vi "Append schedule.vi"(8 "error in (no error)":errorcluster, 10 "Schedule to append":refnum<class "Schedule.lvclass">, 11 "Schedule in":refnum<class "Schedule.lvclass">) -> (0 "error out":errorcluster, 3 "Schedule out":refnum<class "Schedule.lvclass">)   [LabVIEW 2020, in "TALOS.lvlib" / "Run Utilities.lvlib" / "Schedule.lvclass"]
doc: "Combine two schedules into one. The VI checks if the last script of the schedule is the same as the first script of the appended one. If so, it combines two cells into one."
uses:
  Schedule.lvclass
  Cell/Schedule Cell.lvclass
  Schedule.lvclass/Schedule.ctl
  995fc32b-001c-43f1-ab01-1b4acc13e53d.vi
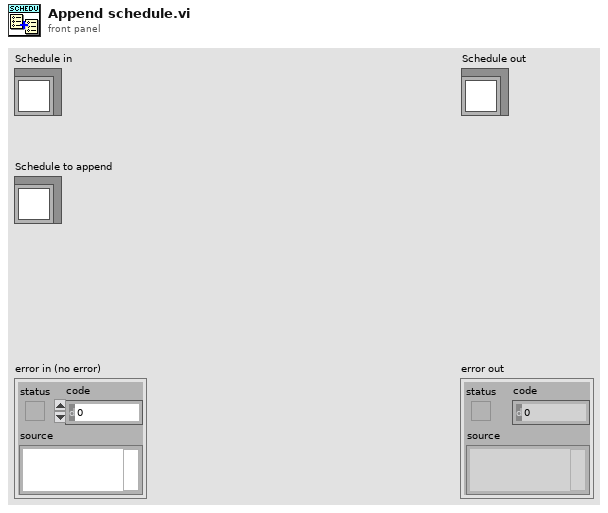
[diagram p1: front panel]
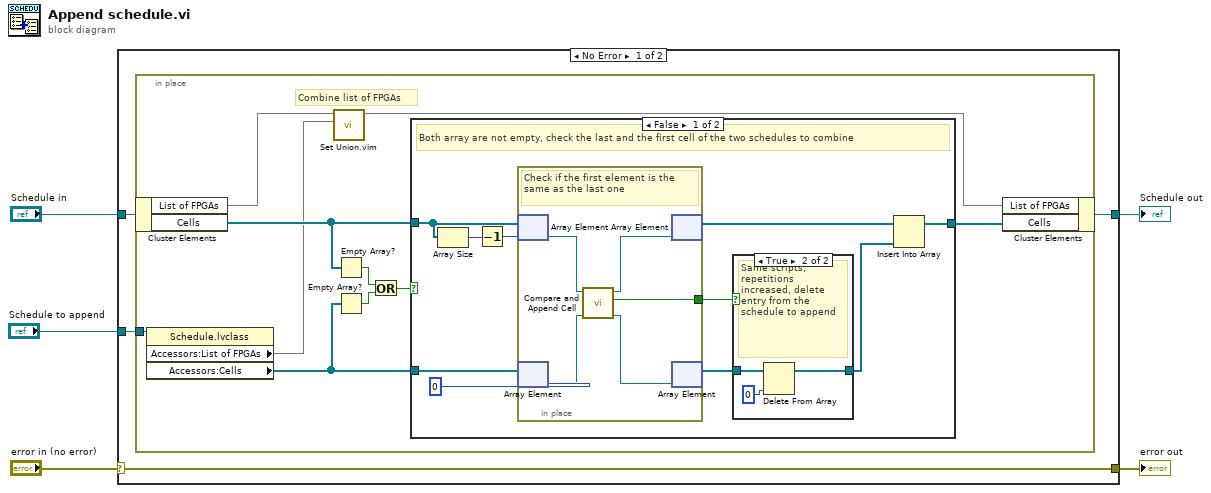
[diagram p0: block diagram]
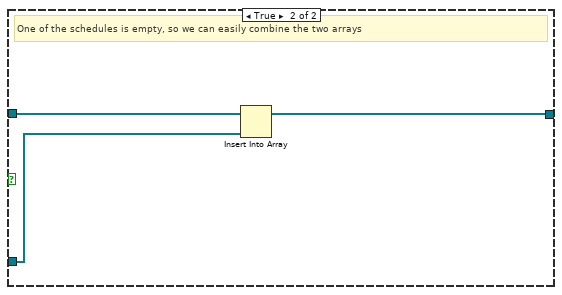
[diagram p3: hidden frame]
diagram:
  n1 = case shown="No Error" "error in (no error)" {
    selector: "error in (no error)" -> [w9 w43]
    tunnel: [w9 w43] -> w4
    tunnel: [w6 w42] -> w2
    tunnel: "Schedule in" -> [w7 w42]
    tunnel: "Schedule to append" -> [w8 _]
    frame No Error {
      n2 = in-place {
        in-place-border: w8 -> [w19]
        # "Combine list of FPGAs"
        n3 = in-place-cluster #1(w7) -> ("List of FPGAs"=w12:set{string}, "Cells"=w18:refnum<class "Schedule Cell.lvclass">[])
        n4 = property class="Schedule.lvclass"(reference=w19) -> ("Accessors:List of FPGAs"=w11:set{string}, "Accessors:Cells"=w16:refnum<class "Schedule Cell.lvclass">[])  [unwired: 1 in, 2 out]
        n5 = call "Set Union.vim"("set 2"=w11, "set 1"=w12) -> ("union"=w10:set{string})  [unwired: 9 in]
        n6 = Empty Array?(array=w18) -> (empty?=w15:bool)
        n7 = Empty Array?(array=w16) -> (empty?=w14:bool)
        n8 = Or(x=w15, y=w14) -> (x .or. y?=w13:bool)
        n9 = case shown="False" w13 {
          tunnel: [w20 w39] -> w17
          tunnel: w18 -> [w29 w41]
          tunnel: w16 -> [w28 w40]
          frame False {
            # "Both array are not empty, check the last and the first cell of the two schedules to combine"
            n10 = Array Size(array=w29) -> (size(s)=w27:i32)
            n11 = Decrement(x=w27) -> (x-1=w26:i32)
            n12 = in-place {
              in-place-border: [w32] -> w24
              # "Check if the first element is the same as the last one"
              n13 = in-place-array #2(w29, w26) -> (w31:refnum<class "Schedule Cell.lvclass">)
              n14 = in-place-array #3(w28, 0) -> (w30:refnum<class "Schedule Cell.lvclass">)
              n15 = call-dynamic "Compare and Append Cell.vi"("Schedule Cell B in"=w30, "Schedule Cell A in"=w31) -> ("Schedule Cell B out"=w33:refnum<class "Schedule Cell.lvclass">, "Cell Updated"=w32:bool, "Schedule Cell A out"=w34:refnum<class "Schedule Cell.lvclass">)  [unwired: 7 in]
              n16 = in-place-array #2(w34) -> (w21:refnum<class "Schedule Cell.lvclass">[])  [unwired: 1 out]
              n17 = in-place-array #3(w33) -> (w23:refnum<class "Schedule Cell.lvclass">[])  [unwired: 1 out]
            }
            n18 = case shown="True" w24 {
              tunnel: w23 -> [w35 w38]
              tunnel: [w35 w36] -> w22
              frame False {
                # "Not the same, do nothing"
              }
              frame True {
                # "Same scripts, repetitions increased, delete entry from the schedule to append"
                n19 = Delete From Array(array=w38, index=0) -> (array with subset deleted=w36:refnum<class "Schedule Cell.lvclass">[])  [unwired: 1 in, 1 out]
              }
            }
            n20 = Insert Into Array(array=w21, new element=w22) -> (w20:refnum<class "Schedule Cell.lvclass">[])  [unwired: 1 in]
          }
          frame True {
            # "One of the schedules is empty, so we can easily combine the two arrays"
            n21 = Insert Into Array(array=w41, new element=w40) -> (w39:refnum<class "Schedule Cell.lvclass">[])  [unwired: 1 in]
          }
        }
        n22 = in-place-cluster #1("List of FPGAs"=w10, "Cells"=w17) -> (w6:refnum<class "Schedule.lvclass">)
      }
    }
    frame Error {
    }
  }
  "error out" <- w4
  "Schedule out" <- w2
